vi "Configure Specific Limit Test.vi"(0 "VISA resource name":refnum<visa-resource-name>, 1 "Enable Limit Test  (T:Enable)":bool=TRUE, 5 "Limit Test Number (2)":u16=2, 7 "Lower Limit (0)":dbl, 9 "Upper Limit (1)":dbl=1.0, 11 "error in (no error)":errorcluster, 12 "Function (0: Volts)":u16(ring) items=["Volts", "Current", "Resistance"]) -> (4 "VISA resource name out":refnum<visa-resource-name>, 15 "error out":errorcluster)   [LabVIEW 2020, in "Keithley 2450.lvlib"]
doc: "Configures limit testing settings, such as the enabling or disabling limit test, setting upper and lower limit."
uses:
  Keithley 2450.lvlib
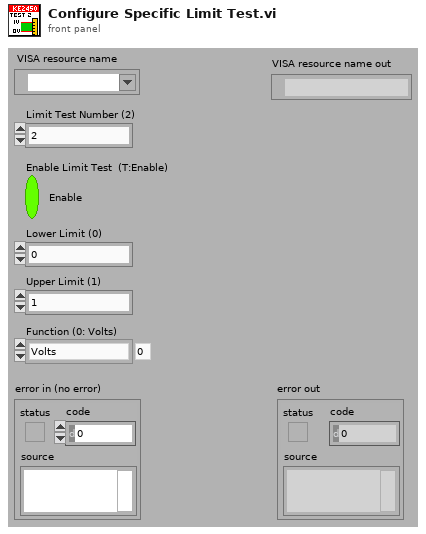
[diagram p1: front panel]
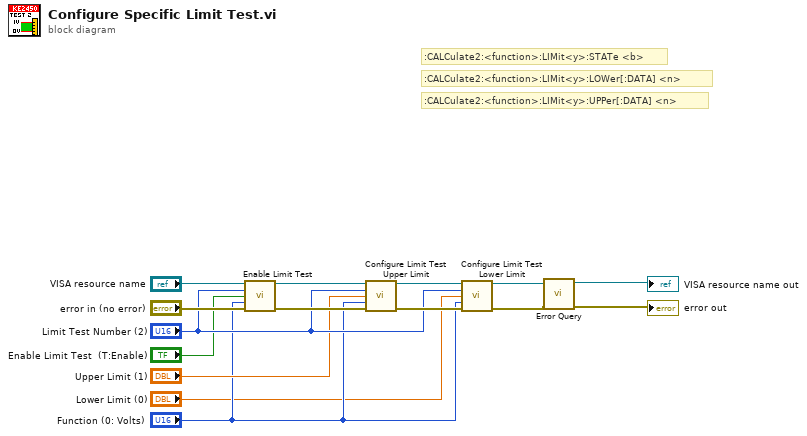
[diagram p0: block diagram]
diagram:
  # ":CALCulate2:<function>:LIMit<y>:UPPer[:DATA] <n>"
  # ":CALCulate2:<function>:LIMit<y>:LOWer[:DATA] <n>"
  # ":CALCulate2:<function>:LIMit<y>:STATe <b>"
  n1 = call "Enable Limit Test.vi"("VISA resource name"="VISA resource name", "Limit Test Number (2)"="Limit Test Number (2)", "Enable Limit Test  (T:Enable)"="Enable Limit Test  (T:Enable)", "Function (0: Volts)"="Function (0: Volts)", "error in (no error)"="error in (no error)") -> ("VISA resource name out"=w11:refnum<visa-resource-name>, "error out"=w14:errorcluster)  [unwired: 9 in]
  n2 = call "Configure Limit Test Upper Limit.vi"("VISA resource name"=w11, "Limit Test Number (1)"="Limit Test Number (2)", "Upper Limit (1)"="Upper Limit (1)", "Function (0: Volts)"="Function (0: Volts)", "error in (no error)"=w14) -> ("VISA resource name out"=w10:refnum<visa-resource-name>, "error out"=w13:errorcluster)  [unwired: 9 in]
  n3 = call "Configure Limit Test Lower Limit.vi"("VISA resource name"=w10, "Limit Test Number (1)"="Limit Test Number (2)", "Lower Limit (-1.0)"="Lower Limit (0)", "Function (0: Volts)"="Function (0: Volts)", "error in (no error)"=w13) -> ("VISA resource name out"=w4:refnum<visa-resource-name>, "error out"=w1:errorcluster)  [unwired: 9 in]
  n4 = call "Error Query.vi"("error in (no error)"=w1, "VISA resource name"=w4) -> ("error out"=→"error out":errorcluster, "VISA resource name out"=→"VISA resource name out":refnum<visa-resource-name>)  [unwired: 6 in, 2 out]
